vi "AprilTag16h5Codes.vi"() -> (0 "Codes":i64[](array[numeric])=[8987, 11941, 13418, 17849, 31142, 32619, -19624, -6331, -423, 5485, 14347, -3925, 3460, 18230, -29582, -20720, 2364, -27724, -23293, 18063, -7881, 22421, -8382, 7197, -5668, 29613, -21153, -10960, 1994, -20690] format="%.0x", 1 "Layout":string)   [LabVIEW 2020, in "feature_detection.lvlib"]
uses:
  feature_detection.lvlib
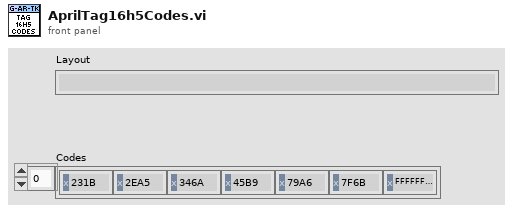
[diagram p1: front panel]
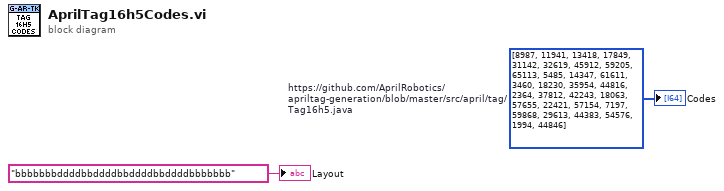
[diagram p0: block diagram]
diagram:
  w2 = i32[] [8987, 11941, 13418, 17849, 31142, 32619, 45912, 59205, 65113, 5485, 14347, 61611, 3460, 18230, 35954, 44816, 2364, 37812, 42243, 18063, 57655, 22421, 57154, 7197, 59868, 29613, 44383, 54576, 1994, 44846]  # https://github.com/AprilRobotics/apriltag-generation/blob/master/src/april/tag/Tag16h5.java
  "Codes" <- w2
  "Layout" <- "bbbbbbbddddbbddddbbddddbbddddbbbbbbb" ("Layout")
